vi "MagBoard_Monitor_n64_v2.vi"() -> ()   [LabVIEW 2016]
doc: "This example performs writes and reads on a serial port, as directed by the user. You can press the Write and Read buttons, and change the Read Count, while the example is running.\n\nThe parameters set for the serial port must match the parameters of the connected instrument or device. In this example, the Read Count parameter specifies the number of bytes that the serial port reads. If there were more bytes at the port than the specified number, those bytes would not be read. If there were less bytes at the port than the specified number, you would receive a timeout error.\n\nThis example expands upon the flow control options for XON and XOFF, allowing the user to choose those control characters. Also, the user can enable or disable a termination character. Some devices require a termination character in order to identify the end of command strings. Some devices send a termination character to signify the end of data to be read. This example shows how you can end the Read operation once a termination character is detected in the buffer and/or append a termination character at the end of the Write data."
uses:
  <vilib>/Native 3D Graph/xcontrol/3DPC_SurfacePlot.xctl
  <vilib>/Native 3D Graph/classes/Line/Line.lvclass
  <vilib>/Instr/_visa.llb/VISA Configure Serial Port (Instr).vi
panel:
  in  "File Progress":dbl(slide) scale=0.0..1.0
  out "Packet OK?":bool=TRUE
  in  "Tab Control":T1(tab)=enum."Basic Data"
  in  "Save Data?":bool
  in  "File Save Path":path
  in  "VISA resource name":refnum<visa-resource-name>="COM11"
  in  "Serial Settings":T2={"baud rate"=115200, "data bits"=8, "parity"=enum."None", "stop bits"=10, "flow control"=0} {"flow control" items=["None"=0, "XON/XOFF"=1, "RTS/CTS"=2, "DTR/DSR"=4]; "stop bits" items=["1.0"=10, "1.5"=15, "2.0"=20]; "data bits" min=5 max=8 step=1; "baud rate" items=["75"=75, "110"=110, "134"=134, "150"=150, "300"=300, "600"=600, "1200"=1200, "1800"=1800, "2400"=2400, "4800"=4800, "7200"=7200, "9600"=9600, "14400"=14400, "19200"=19200, "28800"=28800, "38400"=38400, "56000"=56000, "57600"=57600, "115200"=115200, "128000"=128000, "230400"=230400]}
  in  "XON/XOFF Characters":T3={"XON"=enum."DC1", "XOFF"=enum."DC3"}
  in  "Termination Character":u8=10 format="%.0x"
  in  "Row LEngth":i32=8
  in  "No. Nodes":i32=64
  in  "milliseconds to wait":u32=25
  in  "Data Source":T4(ring)
  in  "File dT":u32=50
  in  "Rows":i32=8
  in  "Cols":i32=8
  in  "XY Spacing":dbl=20.0 format="%#_13g"
  out "read buffer":string
  out "Serial Settings:Number of Bytes at Serial Port":u32
  out "error out":errorcluster
  out "Sensor Nodes Returned":i32=384
  in  "Node to plot":i32=4
  out "B Measure Chart":T5(graph)
  out "Time":u32=427420
  out "Sensor Readings":dbl[][](array[numeric])=[[-533.0, -111.0, 239.0], [-402.0, 166.0, 184.0], [-184.0, 154.0, 29.0], [-106.0, 74.0, 11.0], [-532.0, -109.0, 246.0], [-398.0, 164.0, 175.0], [-205.0, 152.0, 32.0], [-119.0, 65.0, 9.0], [-529.0, -110.0, 242.0], [-408.0, 166.0, 184.0], [-198.0, 158.0, 27.0], [-108.0, 61.0, 6.0], [-539.0, -106.0, 240.0], [-407.0, 158.0, 183.0], [-191.0, 156.0, 28.0], [-113.0, 73.0, 15.0], [816.0, -260.0, 842.0], [539.0, 512.0, 512.0], [156.0, 425.0, 83.0], [13.0, 142.0, -72.0], [816.0, -262.0, 840.0], [528.0, 520.0, 512.0], [162.0, 425.0, 83.0], [13.0, 137.0, -84.0], [809.0, -260.0, 840.0], [538.0, 520.0, 504.0], [162.0, 432.0, 72.0], [13.0, 136.0, -84.0], [809.0, -260.0, 846.0], [538.0, 508.0, 512.0], [158.0, 435.0, 72.0], [19.0, 136.0, -79.0], [346.0, -168.0, 14.0], [287.0, -68.0, 19.0], [161.0, -34.0, 4.0], [70.0, -44.0, -7.0], [345.0, -191.0, 19.0], [279.0, -40.0, 8.0], [167.0, -16.0, 12.0], [72.0, -23.0, 2.0], [341.0, -190.0, 17.0], [285.0, -46.0, 9.0], [149.0, -15.0, 6.0], [54.0, -40.0, -2.0], [375.0, -201.0, 19.0], [282.0, -51.0, 10.0], [135.0, -37.0, 6.0], [81.0, -57.0, -12.0], [-80.0, -193.0, -48.0], [-73.0, -136.0, -12.0], [-5.0, -122.0, -31.0], [-19.0, -118.0, -17.0], [-118.0, -187.0, -48.0], [-73.0, -115.0, -22.0], [1.0, -113.0, -27.0], [-20.0, -111.0, -8.0], [-99.0, -184.0, -40.0], [-62.0, -145.0, -17.0], [0.0, -113.0, -37.0], [-7.0, -117.0, -15.0], [-126.0, -184.0, -50.0], [-72.0, -115.0, -14.0], [-4.0, -114.0, -25.0], [-29.0, -116.0, -14.0]]
  in  "Reset":bool=TRUE
  in  "Tare":bool=TRUE
  out "offset (in bytes)":i64
  out "3D Graph":refnum<class "Base Datatype.lvclass">[](xcontrol)
  in  "XYZ Gain":dbl[](array[numeric])=[0.01, 0.01, 0.1]
  in  "Stop Constant":bool
  in  "Stop Serial":bool
  in  "Stop file":bool
  # "0xA is equivalent to a '\\n' character, which is a line feed."
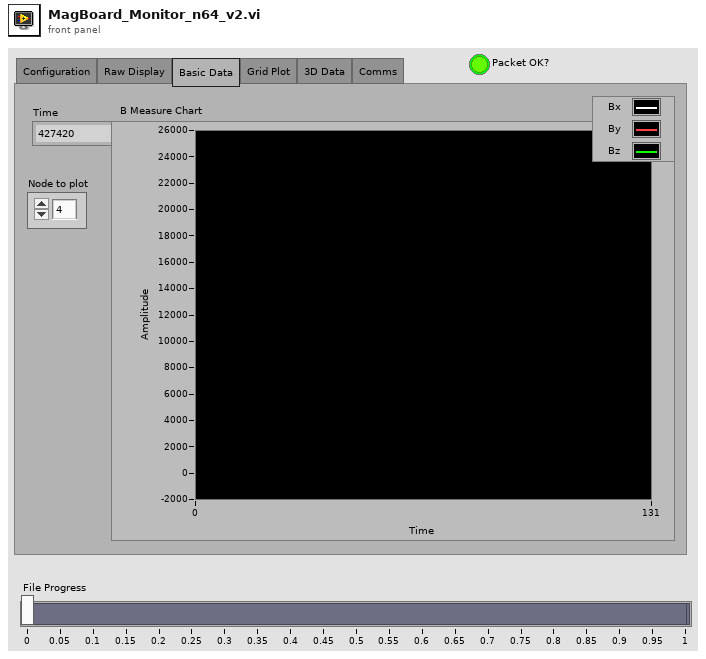
[diagram p1: front panel]
types:
  T1 = enum32{"Configuration", "Raw Display", "Basic Data", "Grid Plot", "3D Data", "Comms"}
  T2 = cluster{"baud rate":u32, "data bits":u16, "parity":enum16{"None", "Odd", "Even", "Mark", "Space"}, "stop bits":u16, "flow control":u16}
  T3 = cluster{"XON":enum16{"NUL", "SOH", "STX", "ETX", "EOT", "ENQ", "ACK", "BEL", "BS", "HT", "LF", "VT", "FF", "CR", "SO", "SI", "DLE", "DC1", "DC2", "DC3", "DC4", "NAK", "SYN", "ETB", "CAN", "EM", "SUB", "ESC", "FS", "GS", "RS", "US", "SP", "!", "\"", "#", "$", "%", "&", "'", "(", ")", "*", "+", ",", "- (-)", ".", "/", "0", "1", "2", "3", "4", "5", "6", "7", "8", "9", ":", ";", "<", "=", ">", "?", "@", "A", "B", "C", "D", "E", "F", "G", "H", "I", "J", "K", "L", "M", "N", "O", "P", "Q", "R", "S", "T", "U", "V", "W", "X", "Y", "Z", "[", "\\", "]", "^", "_", "`", "a", "b", "c", "d", "e", "f", "g", "h", "i", "j", "k", "l", "m", "n", "o", "p", "q", "r", "s", "t", "u", "v", "w", "x", "y", "z", "{", "|", "}", "~"}, "XOFF":enum16{"NUL", "SOH", "STX", "ETX", "EOT", "ENQ", "ACK", "BEL", "BS", "HT", "LF", "VT", "FF", "CR", "SO", "SI", "DLE", "DC1", "DC2", "DC3", "DC4", "NAK", "SYN", "ETB", "CAN", "EM", "SUB", "ESC", "FS", "GS", "RS", "US", "SP", "!", "\"", "#", "$", "%", "&", "'", "(", ")", "*", "+", ",", "- (-)", ".", "/", "0", "1", "2", "3", "4", "5", "6", "7", "8", "9", ":", ";", "<", "=", ">", "?", "@", "A", "B", "C", "D", "E", "F", "G", "H", "I", "J", "K", "L", "M", "N", "O", "P", "Q", "R", "S", "T", "U", "V", "W", "X", "Y", "Z", "[", "\\", "]", "^", "_", "`", "a", "b", "c", "d", "e", "f", "g", "h", "i", "j", "k", "l", "m", "n", "o", "p", "q", "r", "s", "t", "u", "v", "w", "x", "y", "z", "{", "|", "}", "~"}}
  T4 = enum16{"Serial", "Bluetooth", "Data File", "Constant"}
  T5 = cluster{"Node XYZ List[0]":dbl, "Node XYZ List[1]":dbl, "Node XYZ List[2]":dbl}
  T6 = enum16{"open", "replace", "create", "open or create", "replace or create", "replace or create with confirmation"}
  T7 = enum16{"NUL", "SOH", "STX", "ETX", "EOT", "ENQ", "ACK", "BEL", "BS", "HT", "LF", "VT", "FF", "CR", "SO", "SI", "DLE", "DC1", "DC2", "DC3", "DC4", "NAK", "SYN", "ETB", "CAN", "EM", "SUB", "ESC", "FS", "GS", "RS", "US", "SP", "!", "\"", "#", "$", "%", "&", "'", "(", ")", "*", "+", ",", "- (-)", ".", "/", "0", "1", "2", "3", "4", "5", "6", "7", "8", "9", ":", ";", "<", "=", ">", "?", "@", "A", "B", "C", "D", "E", "F", "G", "H", "I", "J", "K", "L", "M", "N", "O", "P", "Q", "R", "S", "T", "U", "V", "W", "X", "Y", "Z", "[", "\\", "]", "^", "_", "`", "a", "b", "c", "d", "e", "f", "g", "h", "i", "j", "k", "l", "m", "n", "o", "p", "q", "r", "s", "t", "u", "v", "w", "x", "y", "z", "{", "|", "}", "~"}
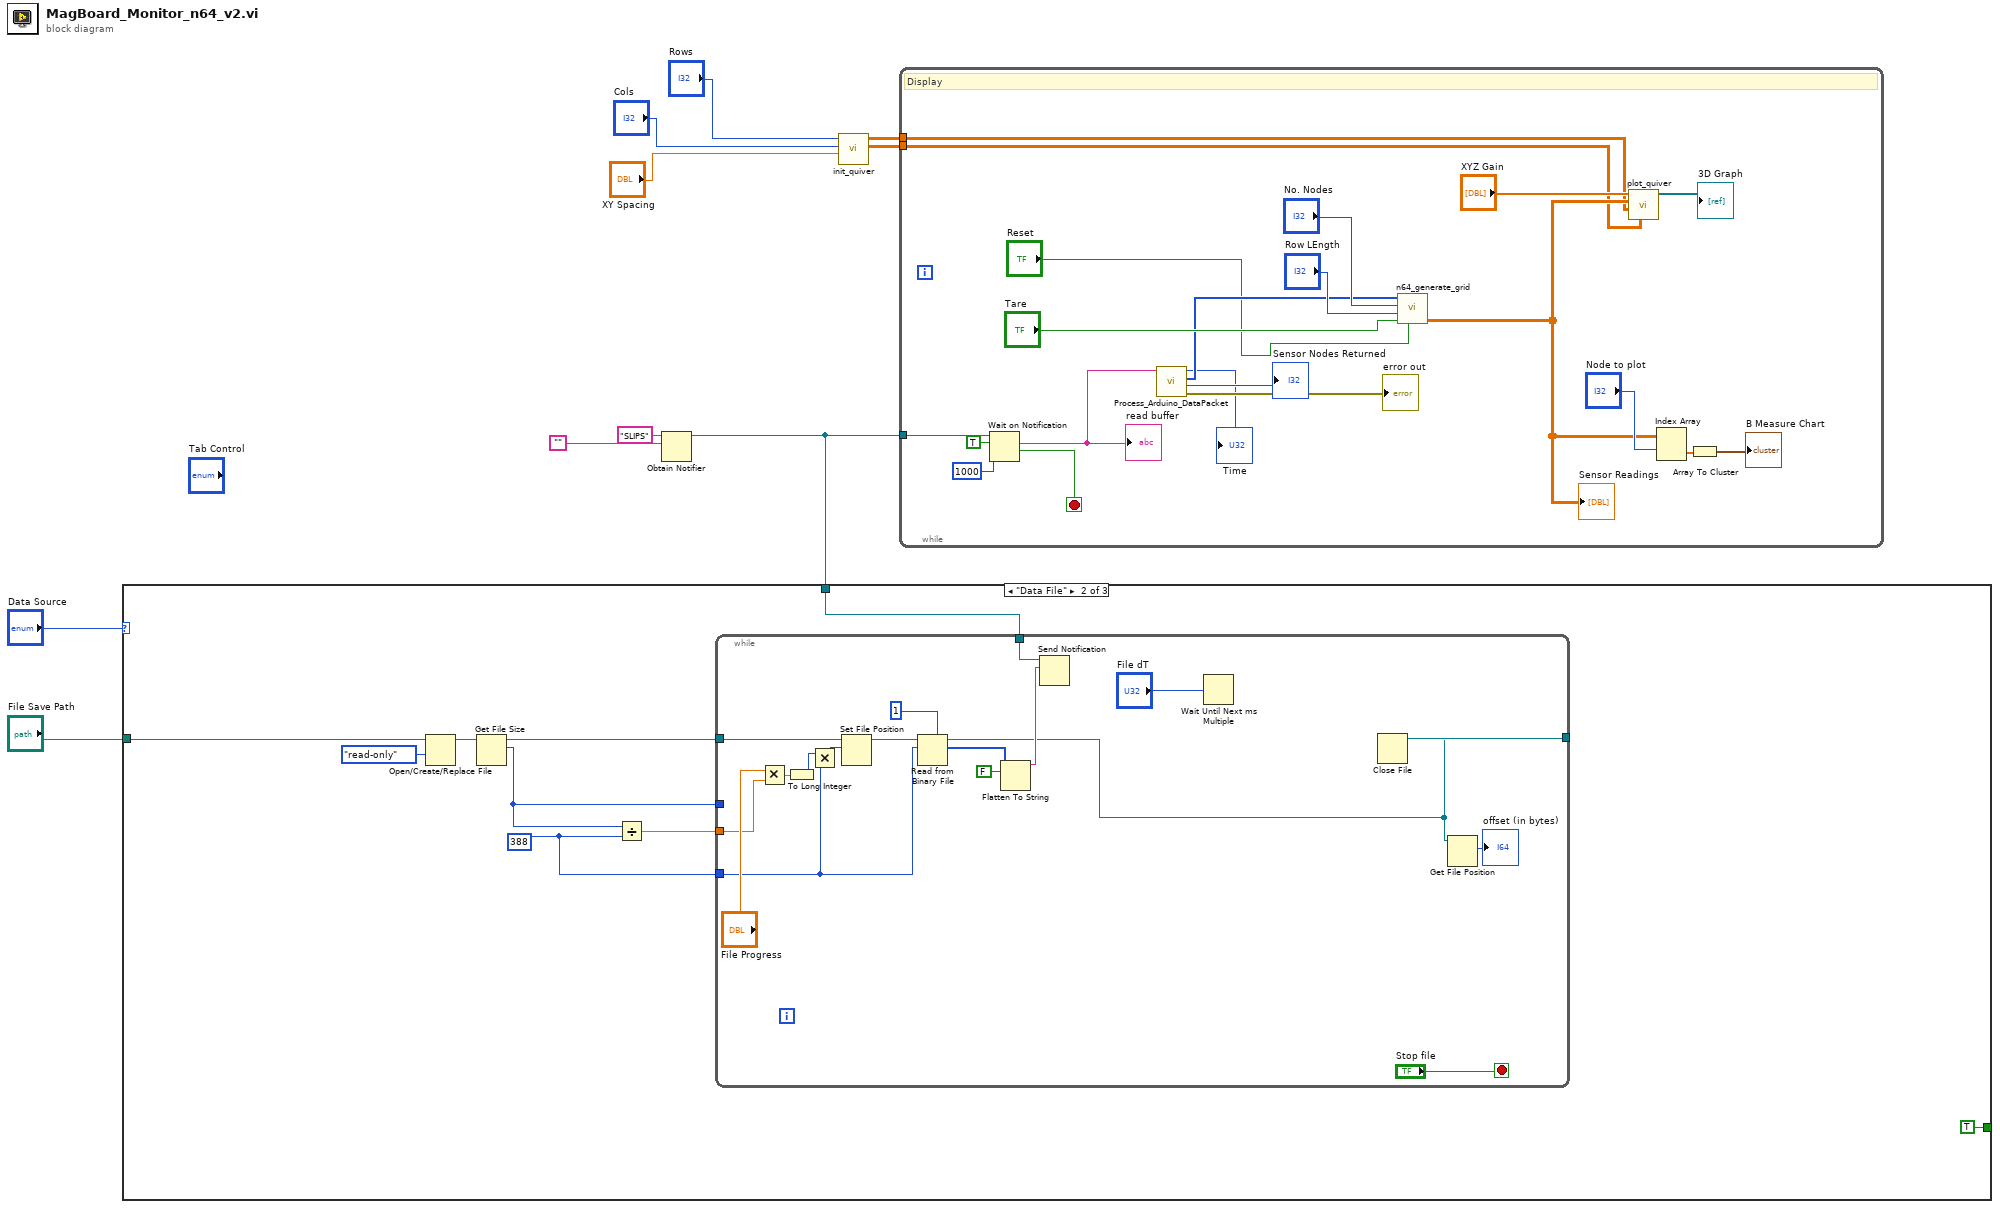
[diagram p0: block diagram]
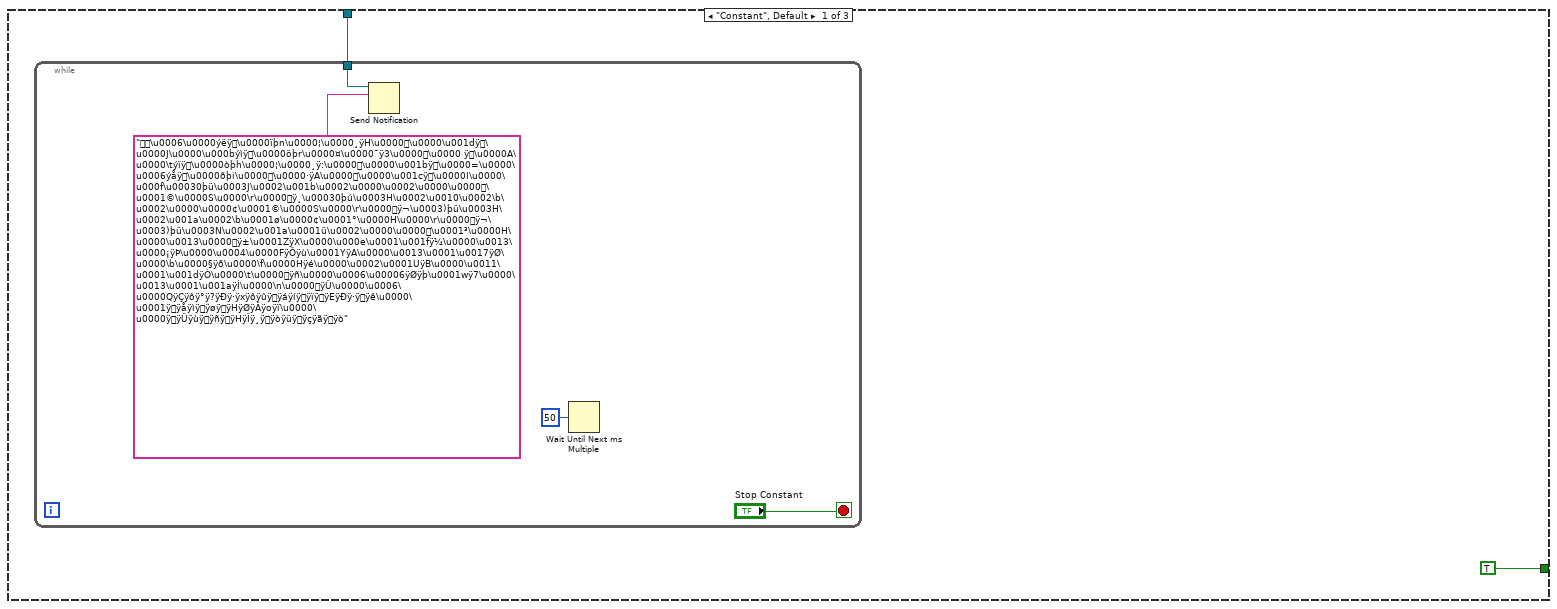
[diagram p2: hidden frame]
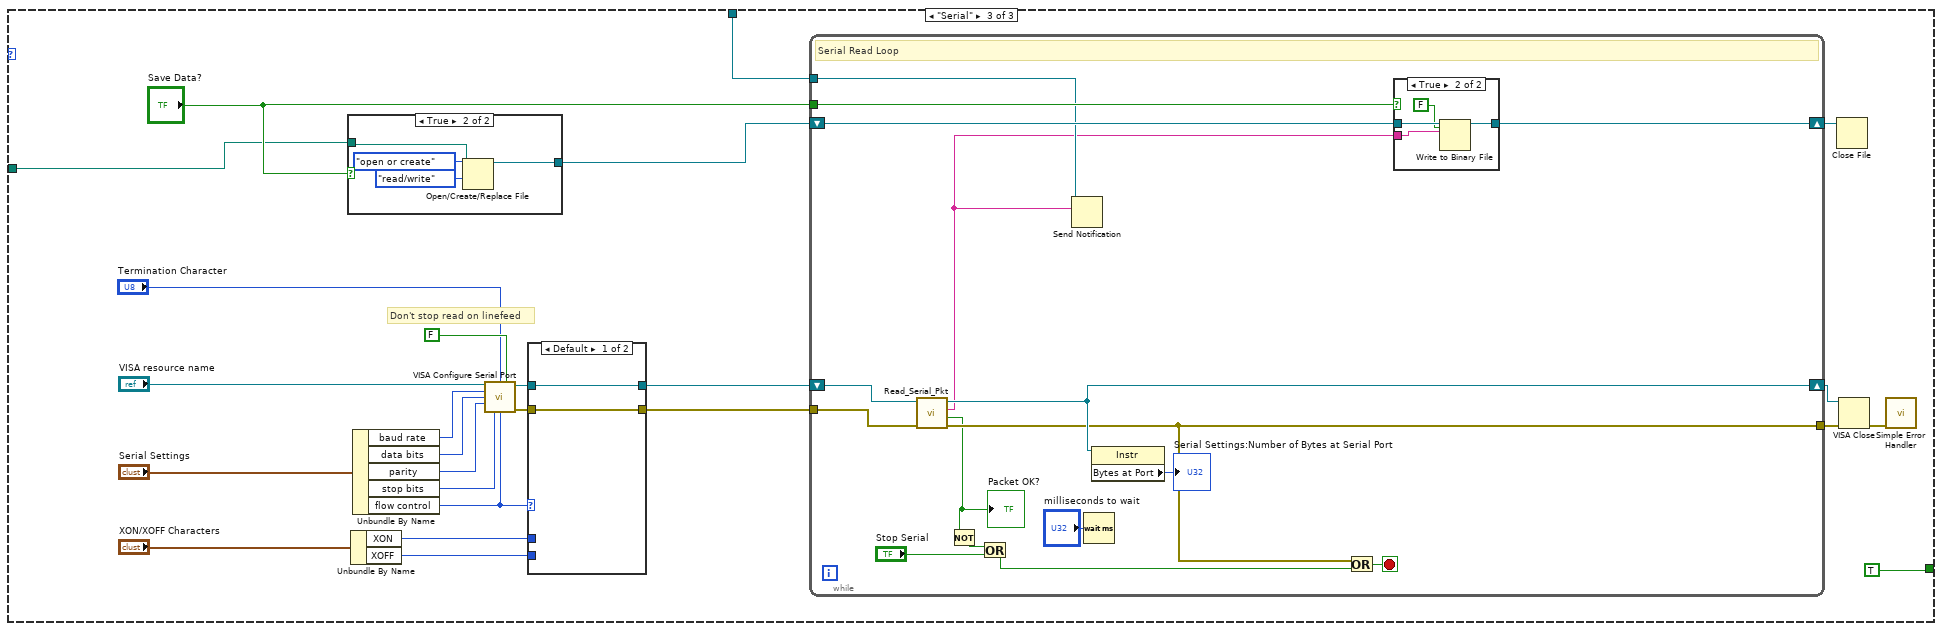
[diagram p3: hidden frame]
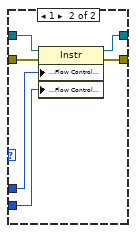
[diagram p4: hidden frame]
diagram:
  n1 = Obtain Notifier(name (unnamed)="SLIPS", notification data type="") -> (notifier out=w10:refnum<notifier>)  [unwired: 2 in, 2 out]
  n2 = case shown="\"Data File\"" "Data Source" {
    tunnel: w10 -> [w12 w26 w60]
    tunnel: [TRUE ("Stop") TRUE ("Stop") TRUE ("Stop")] -> _
    tunnel: "File Save Path" -> [_ w23 w44]
    frame "Constant", Default {
      n3 = while {
        tunnel: w12 -> [w16]
        stop <- "Stop Constant" stop-if-true
        n4 = Send Notification(notification="\u0006\u0000ýëÿ\u0000ïþn\u0000¦\u0000¸ÿH\u0000\u0000\u001dÿ\u0000J\u0000\u000býìÿ\u0000öþr\u0000¤\u0000¯ÿ3\u0000\u0000 ÿ\u0000A\u0000\týïÿ\u0000òþh\u0000¦\u0000¸ÿ:\u0000\u0000\u001bÿ\u0000=\u0000\u0006ýåÿ\u0000ðþi\u0000\u0000·ÿA\u0000\u0000\u001cÿ\u0000I\u0000\u000f\u00030þü\u0003J\u0002\u001b\u0002\u0000\u0002\u0000\u0000\u0001©\u0000S\u0000\r\u0000ÿ¸\u00030þú\u0003H\u0002\u0010\u0002\b\u0002\u0000\u0000¢\u0001©\u0000S\u0000\r\u0000ÿ¬\u0003)þü\u0003H\u0002\u001a\u0002\b\u0001ø\u0000¢\u0001°\u0000H\u0000\r\u0000ÿ¬\u0003)þü\u0003N\u0002\u001a\u0001ü\u0002\u0000\u0000\u0001³\u0000H\u0000\u0013\u0000ÿ±\u0001ZÿX\u0000\u000e\u0001\u001fÿ¼\u0000\u0013\u0000¡ÿÞ\u0000\u0004\u0000FÿÔÿù\u0001YÿA\u0000\u0013\u0001\u0017ÿØ\u0000\b\u0000§ÿð\u0000\f\u0000Hÿé\u0000\u0002\u0001UÿB\u0000\u0011\u0001\u001dÿÒ\u0000\t\u0000ÿñ\u0000\u0006\u00006ÿØÿþ\u0001wÿ7\u0000\u0013\u0001\u001aÿÍ\u0000\n\u0000ÿÛ\u0000\u0006\u0000QÿÇÿôÿ°ÿ?ÿÐÿ·ÿxÿôÿûÿÿáÿíÿÿïÿÿEÿÐÿ·ÿÿê\u0000\u0001ÿÿåÿìÿÿøÿÿHÿØÿÂÿoÿï\u0000\u0000ÿÿÛÿùÿÿñÿÿHÿÎÿ¸ÿÿòÿüÿÿçÿãÿÿò" ("read buffer"), notifier=w16) -> ()  [unwired: 1 in, 2 out]
        n5 = Wait Until Next ms Multiple(millisecond multiple=u32 50) -> ()  [unwired: 1 out]
      }
    }
    frame "Data File" {
      w18 = 388 ("count (1)")
      n6 = Open/Create/Replace File(file path (use dialog)=w23, access (0:read/write)=enum16{"read/write", "read-only", "write-only"}."read-only") -> (refnum out=w21:refnum<file>)  [unwired: 4 in, 2 out]
      n7 = Get File Size(file=w21) -> (refnum out=w20:refnum<file>, size (in bytes)=w17:i64)  [unwired: 1 in, 1 out]
      n8 = Divide(x=w17, y=w18) -> (x/y=w19:dbl)
      n9 = while {
        tunnel: w26 -> [w43]
        tunnel: w20 -> [w35]
        tunnel: [w32] -> w24
        tunnel: w19 -> [w31]
        tunnel: w18 -> [w27]
        tunnel: w17 -> [_]
        stop <- "Stop file" stop-if-true
        n10 = Multiply(x="File Progress", y=w31) -> (x*y=w30:dbl)
        n11 = To Long Integer(number=w30) -> (32bit integer=w28:i32)
        n12 = Multiply(x=w28, y=w27) -> (x*y=w29:i32)
        n13 = Set File Position(offset (in bytes) (0)=w29, refnum=w35) -> (refnum out=w34:refnum<file>)  [unwired: 2 in, 1 out]
        n14 = Read from Binary File(5:u8 1 ("count (1)"), 10:w27, 11:w34) -> (2:w40:u8[], 3:w32:refnum<file>)  [unwired: 3 in, 2 out]
        n15 = Flatten To String(anything=w40, prepend array or string size? (T)=FALSE) -> (data string=w39:string)  [unwired: 2 in, 2 out]
        n16 = Send Notification(notification=w39, notifier=w43) -> ()  [unwired: 1 in, 2 out]
        n17 = Wait Until Next ms Multiple(millisecond multiple="File dT") -> ()  [unwired: 1 out]
        n18 = Get File Position(7:w32) -> (2:→"offset (in bytes)":i64)  [unwired: 1 in, 2 out]
      }
      n19 = Close File(refnum=w24) -> ()  [unwired: 1 in, 2 out]
    }
    frame "Serial" {
      # "Don't stop read on linefeed"
      n20 = case shown="True" "Save Data?" {
        tunnel: w44 -> [_ w80]
        tunnel: [_ w78] -> w63
        frame False {
        }
        frame True {
          n21 = Open/Create/Replace File(file path (use dialog)=w80, operation (0:open)=T6."open or create", access (0:read/write)=enum16{"read/write", "read-only", "write-only"}."read/write") -> (refnum out=w78:refnum<file>)  [unwired: 3 in, 2 out]
        }
      }
      n22 = Unbundle By Name("XON/XOFF Characters") -> ("XON"=w48:T7, "XOFF"=w47:T7)
      n23 = Unbundle By Name("Serial Settings") -> ("baud rate"=w52:u32, "data bits"=w53:u16, "parity"=w54:enum16{"None", "Odd", "Even", "Mark", "Space"}, "stop bits"=w55:u16, "flow control"=w49:u16)
      n24 = call-poly "VISA Configure Serial Port"("VISA resource name"="VISA resource name", "termination char\n(0xA = '\\n' = LF)"="Termination Character", "Enable Termination\nChar (T)"=FALSE ("End Read on Termination Character?"), "baud rate (9600)"=w52, "data bits (8)"=w53, "parity (0:none)"=w54, "stop bits (10: 1 bit)"=w55, "flow control (0:none)"=w49) -> ("VISA resource name out"=w56:refnum<visa-resource-name>, "error out"=w57:errorcluster)  [unwired: 2 in, 4 out]
      n25 = case shown="Default" w49 {
        tunnel: [w69 w76] -> w64
        tunnel: [w70 w75] -> w65
        tunnel: w57 -> [w69 w74]
        tunnel: w56 -> [w70 w73]
        tunnel: w48 -> [_ w72]
        tunnel: w47 -> [_ w71]
        frame Default {
        }
        frame 1 {
          n26 = property class="Instr"(reference=w73, error in=w74, "Serial Settings:Flow Control XON Character"=w72, "Serial Settings:Flow Control XOFF Character"=w71) -> (reference out=w75:refnum<visa-resource-name>, error out=w76:errorcluster)
        }
      }
      n27 = while {
        shift-right: [w92] -> w66
        shift-left: w65 -> [w93]
        tunnel: w64 -> [w94]
        tunnel: [w91] -> w67
        tunnel: "Save Data?" -> [w85]
        shift-right: [w84] -> w61
        shift-left: w63 -> [w86]
        tunnel: w60 -> [w82]
        stop <- w83 stop-if-true
        # "Serial Read Loop"
        n28 = call "Read_Serial_Pkt.vi"("error in"=w94, "VISA resource in"=w93) -> ("error out"=w91:errorcluster, "Packet OK?"=w90:bool, "Data"=w81:string, "VISA resource out"=w92:refnum<visa-resource-name>)  [unwired: 6 in]
        "Packet OK?" <- w90
        n29 = Not(x=w90) -> (.not. x?=w87:bool)
        n30 = Or(x=w87, y="Stop Serial") -> (x .or. y?=w88:bool)
        n31 = Send Notification(notification=w81, notifier=w82) -> ()  [unwired: 1 in, 2 out]
        n32 = Wait (ms)(milliseconds to wait="milliseconds to wait") -> ()  [unwired: 1 out]
        n33 = property class="Instr"(reference=w92) -> ("Bytes at Port"=→"Serial Settings:Number of Bytes at Serial Port":u32)  [unwired: 1 in, 2 out]
        n34 = Or(x=w91, y=w88) -> (x .or. y?=w83:bool)
        n35 = case shown="True" w85 {
          tunnel: w86 -> [_ w100]
          tunnel: w81 -> [_ w99]
          tunnel: [_ w97] -> w84
          frame False {
          }
          frame True {
            n36 = Write to Binary File(file (use dialog)=w100, data=w99, 5:FALSE ("prepend array or string size? (T)")) -> (refnum out=w97:refnum<file>)  [unwired: 3 in, 2 out]
          }
        }
      }
      n37 = Close File(refnum=w61) -> ()  [unwired: 1 in, 2 out]
      n38 = VISA Close(VISA resource name=w66, error in (no error)=w67) -> (error out=w68:errorcluster)
      n39 = call <vilib>:"Simple Error Handler.vi"("error in (no error)"=w68) -> ()  [unwired: 1 in, 8 out]
    }
  }
  n40 = call "init_quiver.vi"("XY Spacing"="XY Spacing", "Cols"="Cols", "Rows"="Rows") -> ("Quiver Data Prealloc"=w1:dbl[][], "Quiver Grid"=w2:dbl[][])  [unwired: 7 in]
  n41 = while {
    tunnel: w10 -> [w111]
    tunnel: w2 -> [w103]
    tunnel: w1 -> [w102]
    stop <- w108 stop-if-true
    # "Display"
    n42 = Wait on Notification(notifier=w111, ignore previous (F)=TRUE, timeout in ms (-1)=1000) -> (notification=w110:string, timed out?=w108:bool)  [unwired: 1 in, 2 out]
    "read buffer" <- w110
    n43 = call "Process_Arduino_DataPacket.vi"("Data Packet"=w110) -> ("error out"=→"error out":errorcluster, "Sensor Packets Returned"=→"Sensor Nodes Returned":i32, "Sensor Readings (Signed)"=w116:i16[], "Time"=→"Time":u32)  [unwired: 7 in]
    n44 = call "n64_generate_grid.vi"("Reset"="Reset", "Tare"="Tare", "Row Length"="Row LEngth", "No. Nodes"="No. Nodes", "Sensor Readings (PACKET)"=w116) -> ("Node XYZ List"=w105:dbl[][])  [unwired: 2 in, 4 out]
    "Sensor Readings" <- w105
    n45 = call "plot_quiver.vi"("Quiver Data Prealloc"=w102, "Quiver Grid"=w103, "Sensor Readings"=w105, "XYZ Gain"="XYZ Gain") -> ("plots out"=→"3D Graph":refnum<class "Base Datatype.lvclass">[])  [unwired: 4 in, 3 out]
    n46 = Index Array(array=w105, index (row)="Node to plot") -> (element=w117:dbl[])  [unwired: 1 in]
    n47 = Array To Cluster(array=w117) -> (cluster=→"B Measure Chart":T5)
  }
